vi "initialise.vi"(10 "depth":u32) -> (3 "on-board buffer out":T1)   [LabVIEW 2010, in "OnBoardBuffer.lvlib"]
uses:
  OnBoardBuffer.lvlib
  OnBoardBuffer.ctl
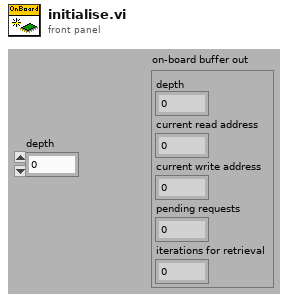
[diagram p1: front panel]
types:
  T1 = typedef "OnBoardBuffer.lvlib/OnBoardBuffer.ctl" = cluster{"depth":u32, "current read address":u32, "current write address":u32, "pending requests":u32, "iterations for retrieval":u32}
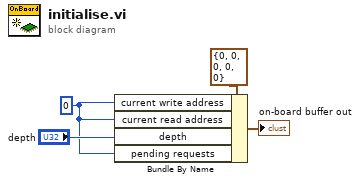
[diagram p0: block diagram]
diagram:
  w1 = u32 0 ("current write address")
  n1 = Bundle By Name(cluster=T1 {"depth"=0, "current read address"=0, "current write address"=0, "pending requests"=0, "iterations for retrieval"=0} ("on-board buffer out"), "current write address"=w1, "current read address"=w1, "depth"="depth", "pending requests"=w1) -> (→"on-board buffer out":T1)
